vi "Main.vi"(11 "Module Admin":refnum<class "Delacor_lib_QMH_Module Admin.lvclass">) -> ()   [LabVIEW 2021, in "Log.lvlib"]
doc: "This template is based off of the Queued Message Handler design pattern and the Queued Message Handler project template that ships with LabVIEW.\n\nThe main difference is that the queue is private to this module and communication between modules is performed via Broadcast and Request events.\n\nRequest events are wrapped in public API methods and are handled in the Event Handling Loop (EHL) of this VI. Any module can register for Broadcast events sent by this module. The EHL generates messages based on user interface actions.\n\nThe Message Handling Loop (MHL) processes messages generated by the EHL, or by other messages. The messages are string values, so new messages can be added easily to the Message Cases case structure in the MHL. Each message cluster can also provide an optional value for Message Data, which is a variant that can be converted to whatever message-specific data is required.\n_____\nBased on DQMH Project Template 7.0.1.1316."
uses:
  Log.lvlib
  <vilib>/Delacor/Delacor QMH/Libraries/Module Admin_class/Delacor_lib_QMH_Module Admin.lvclass
  Module Data--cluster.ctl
  <vilib>/Delacor/Delacor QMH/Libraries/Message Queue_class/Delacor_lib_QMH_Message Queue.lvclass/Delacor_lib_QMH_Message Queue.ctl
  Stop Argument--cluster.ctl
  <vilib>/Delacor/Delacor QMH/Libraries/Module Admin_class/Delacor_lib_QMH_Module Admin.lvclass/Delacor_lib_QMH_Module Admin.ctl
  Log Start Argument--cluster.ctl
  Log Stop Argument--cluster.ctl
  Log Data Argument--cluster.ctl
  <vilib>/Utility/miscctls.llb/LVPointTypeDef.ctl
  <vilib>/Delacor/Delacor QMH/Libraries/Message Queue_class/Delacor_lib_QMH_Enqueue Message (Single).vi
  <vilib>/Delacor/Delacor QMH/Libraries/Module Admin_class/Delacor_lib_QMH_Get External Launch.vi
  <vilib>/Delacor/Delacor QMH/Libraries/Message Queue_class/Delacor_lib_QMH_Message Queue.lvclass
panel:
  out "error out":errorcluster
  out "Status":string
  in  "Simulate MHL Error":bool
  in  "Simulate EHL Error":bool
  # "Other processes communicate with this Module via its Public API (wrappers for its Request Events).\n\nThis Module communicates with other processes via its Broadcast Events.\nAny process that wants to receive these messages can register for this module's Broadcast events."
  # "This template is for the DQMH framework. See the block diagram for more information on how to use this template."
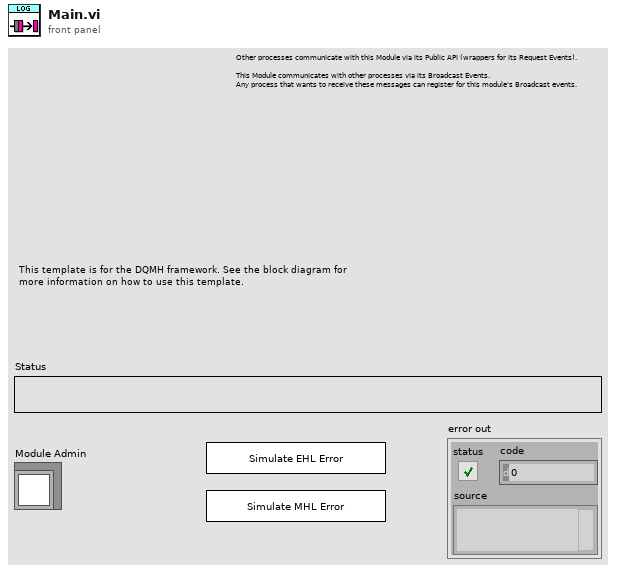
[diagram p1: front panel]
types:
  T1 = typedef "Log.lvlib/Request Events--cluster.ctl" = cluster{"Stop Module":refnum<user-event>, "Show Panel":refnum<user-event>, "Hide Panel":refnum<user-event>, "Get Module Execution Status":refnum<user-event>, "Show Diagram":refnum<user-event>, "Log Start":refnum<user-event>, "Log Stop":refnum<user-event>, "Log Data":refnum<user-event>}
  T2 = typedef "Log.lvlib/Module Data--cluster.ctl" = cluster{"Status":string, "Signal Name":string, "Log Status":bool, "Log Reference":refnum<k34>}
  T3 = enum32{"invalid lock state", "Not Locked", "Locked (No Password)", "Password-protected"}
  T4 = typedef "Log.lvlib/Stop Argument--cluster.ctl" = cluster{"Origin":string, "Exit via Stop Module Req?":bool, "Wait for Module to stop?":bool}
  T5 = typedef "Log.lvlib/Log Start Argument--cluster.ctl" = cluster{"Signal Name":string}
  T6 = typedef "Log.lvlib/Log Stop Argument--cluster.ctl" = cluster{"Boolean":bool}
  T7 = typedef "Log.lvlib/Log Data Argument--cluster.ctl" = cluster{"Signal":waveform(dbl)}
  T8 = typedef "LVPointTypeDef.ctl" = cluster{"Horizontal":i16, "Vertical":i16}
  T9 = enum32{"Invalid", "Standard", "Closed", "Hidden", "Minimized", "Maximized"}
  T10 = enum16{"open", "open or create", "create or replace", "create", "open (read-only)"}
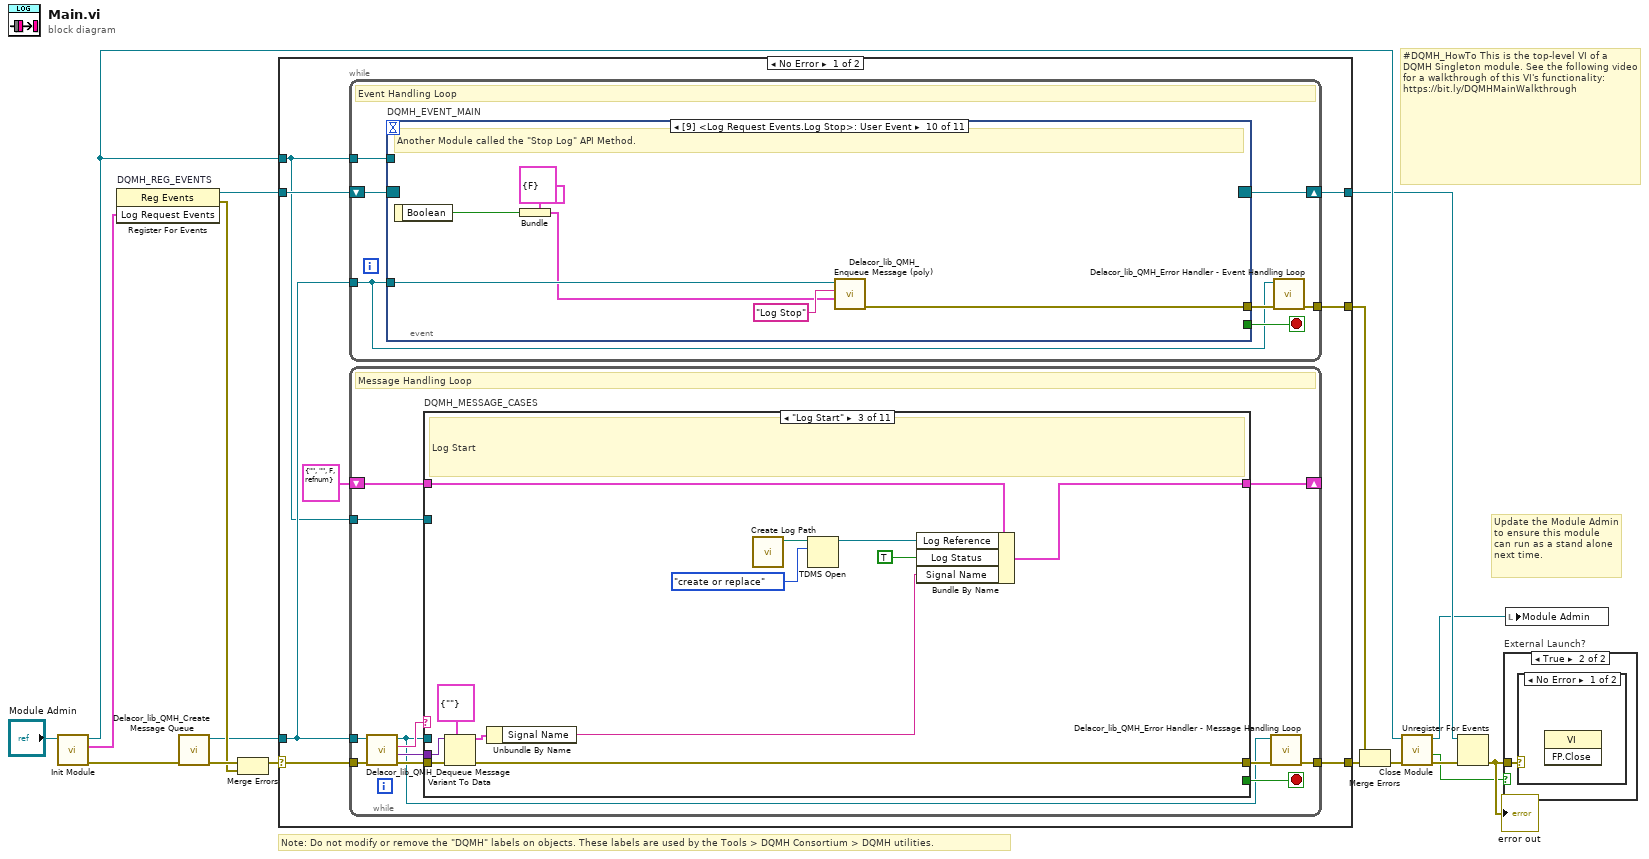
[diagram p0: block diagram]
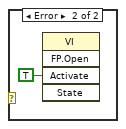
[diagram p3: hidden frame]
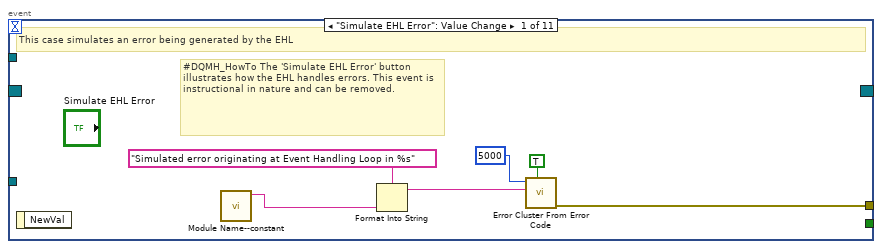
[diagram p4: hidden frame]
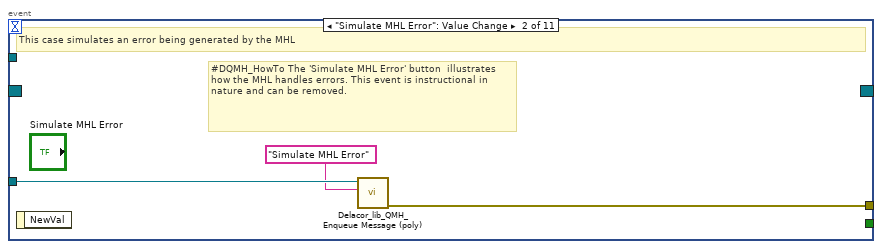
[diagram p5: hidden frame]
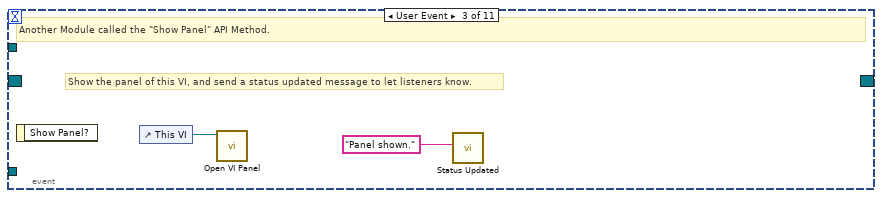
[diagram p6: hidden frame]
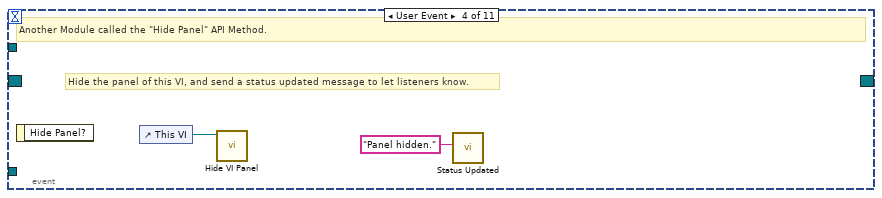
[diagram p7: hidden frame]
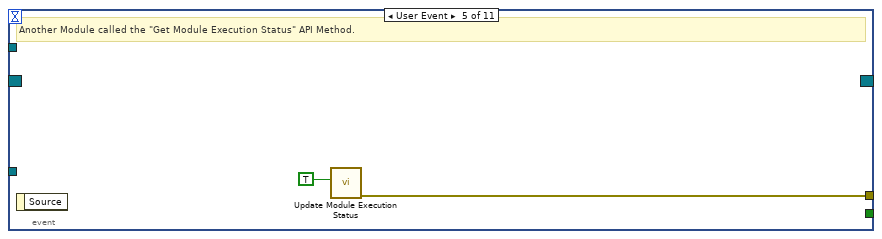
[diagram p8: hidden frame]
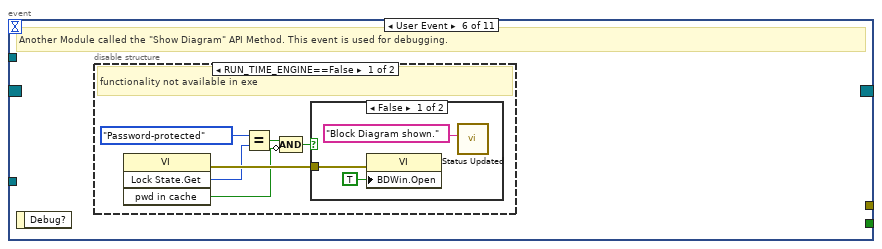
[diagram p9: hidden frame]
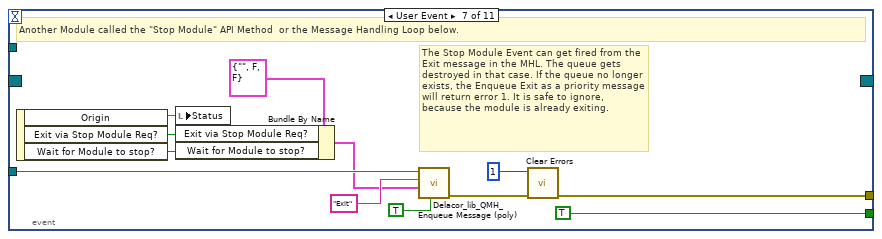
[diagram p12: hidden frame]
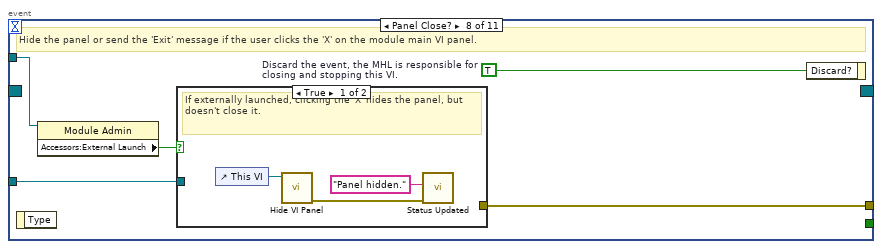
[diagram p13: hidden frame]
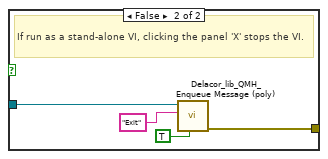
[diagram p14: hidden frame]
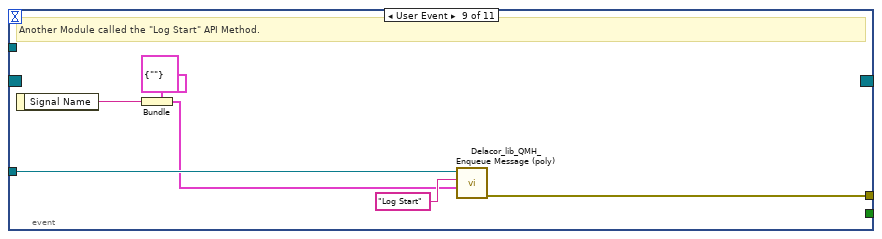
[diagram p15: hidden frame]
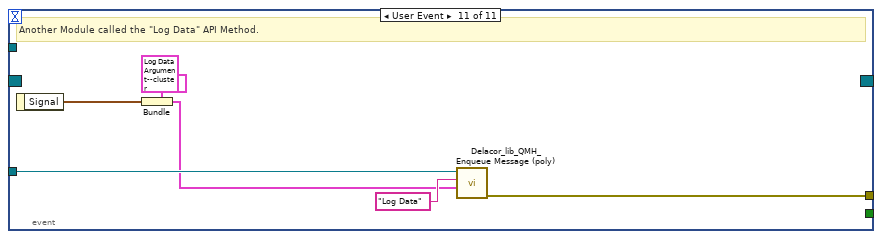
[diagram p16: hidden frame]
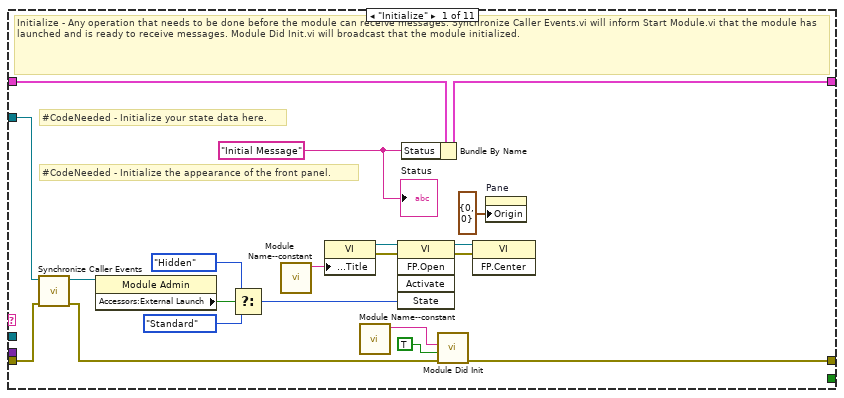
[diagram p17: hidden frame]
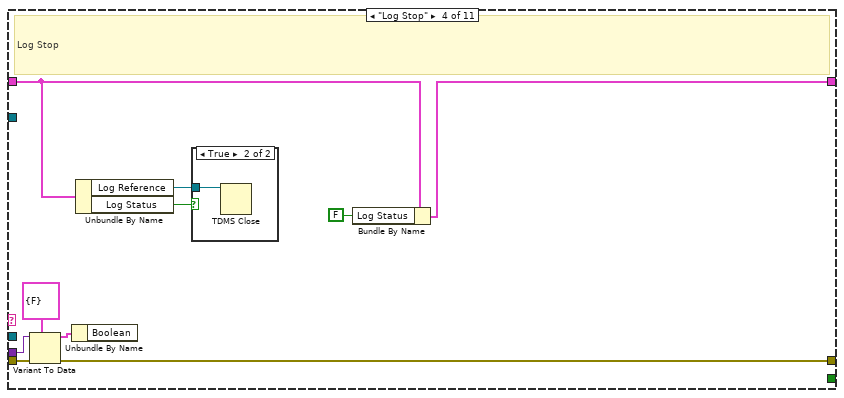
[diagram p19: hidden frame]
diagram:
  # "#DQMH_HowTo This is the top-level VI of a DQMH Singleton module. See the following video for a walkthrough of this VI's functionality: https://bit.ly/DQMHMainWalkthrough"
  # "Note: Do not modify or remove the \"DQMH\" labels on objects. These labels are used by the Tools > DQMH Consortium > DQMH utilities."
  # "Update the Module Admin to ensure this module can run as a stand alone next time."
  n1 = call "Init Module.vi"("Singleton Module Admin in"="Module Admin") -> ("error out"=w16:errorcluster, "Log Request Events"=w5:T1, "Singleton Module Admin out"=w8:refnum<class "Delacor_lib_QMH_Module Admin.lvclass">)  [unwired: 8 in]
  n2 = register-events "DQMH_REG_EVENTS"(w5) -> (reference out=w6:refnum<event-registration>, error out=w9:errorcluster)  [unwired: 2 in]
  n3 = call <vilib>:"Delacor_lib_QMH_Create Message Queue.vi"("error in"=w16) -> ("error out"=w11:errorcluster, "Message Queue"=w4:refnum<class "Delacor_lib_QMH_Message Queue.lvclass">)  [unwired: 9 in]
  n4 = Merge Errors(w11, w9) -> (w10:errorcluster)
  n5 = case shown="No Error" w10 {
    selector: w10 -> [w23 w233]
    tunnel: [w25 w232] -> w17
    tunnel: [w22 w231] -> w7
    tunnel: w6 -> [w20 w231]
    tunnel: w4 -> [w19 w226]
    tunnel: [w24 _] -> w14
    tunnel: w8 -> [w18 w227]
    frame No Error {
      n6 = while {
        tunnel: w19 -> [w26]
        shift-right: [w29] -> w22
        shift-left: w20 -> [w30]
        tunnel: [w31] -> w24
        tunnel: w18 -> [w27]
        stop <- w28 stop-if-true
        # "Event Handling Loop"
        n7 = event "DQMH_EVENT_MAIN" shown="[9] <Log Request Events.Log Stop>: User Event" {
          selector: w30 -> [_ _ _ _ _ _ _ _ _ _ _]
          dyn-events: [_ _ _ _ _ _ _ _ _ _ _] -> w29
          timeout: _ -> [_ _ _ _ _ _ _ _ _ _ _]
          tunnel: [_ _ _ _ _ _ TRUE ("Discard?") _ _ _ _] -> w28
          tunnel: w26 -> [_ w40 _ _ _ _ w64 w71 w86 w92 w98]
          tunnel: [w38 w41 _ _ w47 _ w67 w73 w81 w87 w93] -> w32
          tunnel: w27 -> [_ _ _ _ _ _ _ w70 _ _ _]
          event "Simulate EHL Error": Value Change {
            # "#DQMH_HowTo The 'Simulate EHL Error' button  illustrates how the EHL handles errors. This event is instructional in nature and can be removed."
            # "This case simulates an error being generated by the EHL"
            n8 = event-data() -> ()  [unwired: 1 in, 1 out]
            n9 = call "Module Name--constant.vi"() -> ("Module Name"=w35:string)  [unwired: 11 in]
            n10 = Format Into String(format string="Simulated error originating at Event Handling Loop in %s", w35) -> (resulting string=w36:string)  [unwired: 2 in, 1 out]
            n11 = call <vilib>:"Error Cluster From Error Code.vi"("show call chain? (False)"=TRUE, "error message (\"\")"=w36, "error code (0)"=5000) -> ("error out"=w38:errorcluster)  [unwired: 6 in]
          }
          event "Simulate MHL Error": Value Change {
            # "#DQMH_HowTo The 'Simulate MHL Error' button  illustrates how the MHL handles errors. This event is instructional in nature and can be removed."
            # "This case simulates an error being generated by the MHL"
            n12 = event-data() -> ()  [unwired: 1 in, 1 out]
            n13 = call-poly <vilib>:"Delacor_lib_QMH_Enqueue Message (poly).vi"("Message"="Simulate MHL Error", "Message Queue in"=w40) -> ("error out"=w41:errorcluster)  [unwired: 8 in, 1 out]
          }
          event User Event {
            # "Show the panel of this VI, and send a status updated message to let listeners know."
            # "Another Module called the \"Show Panel\" API Method."
            n14 = event-data() -> ()  [unwired: 1 in, 1 out]
            n15 = control-ref of="This VI"() -> (w43:refnum<vi>)
            n16 = call "Open VI Panel.vi"("VI"=w43) -> ()  [unwired: 10 in, 1 out]
            n17 = call "Status Updated.vi"("Status"="Panel shown." ("format string")) -> ()  [unwired: 10 in, 1 out]
          }
          event User Event {
            # "Hide the panel of this VI, and send a status updated message to let listeners know."
            # "Another Module called the \"Hide Panel\" API Method."
            n18 = event-data() -> ()  [unwired: 1 in, 1 out]
            n19 = control-ref of="This VI"() -> (w45:refnum<vi>)
            n20 = call "Hide VI Panel.vi"("VI"=w45) -> ()  [unwired: 10 in, 1 out]
            n21 = call "Status Updated.vi"("Status"="Panel hidden." ("format string")) -> ()  [unwired: 10 in, 1 out]
          }
          event User Event {
            # "Another Module called the \"Get Module Execution Status\" API Method."
            n22 = event-data() -> ()  [unwired: 1 in, 1 out]
            n23 = call "Update Module Execution Status.vi"("Running?"=TRUE) -> ("error out"=w47:errorcluster)  [unwired: 10 in]
          }
          event User Event {
            # "Another Module called the \"Show Diagram\" API Method. This event is used for debugging."
            n24 = event-data() -> ()  [unwired: 1 in, 1 out]
            n25 = disable-structure shown="RUN_TIME_ENGINE==False" {
              frame condition #0 (active) {
                # "functionality not available in exe"
                n26 = invoke on="Invoke Node" class="VI" method="Lock State.Get"() -> (error out=w53:errorcluster, "Get Lock State"=w52:T3, "pwd in cache"=w49:bool)  [unwired: 4 in, 1 out]
                n27 = Equal?(x=T3."Password-protected", y=w52) -> (x = y?=w50:bool)
                n28 = Compound Arithmetic op=AND(w50, invert w49) -> (w48:bool)
                n29 = case shown="False" w48 {
                  tunnel: w53 -> [w56 _]
                  frame False {
                    n30 = property on="Property Node" class="VI"(error in=w56, "BDWin.Open"=TRUE ("Block Diagram Window:Open")) -> ()  [unwired: 1 in, 2 out]
                    n31 = call "Status Updated.vi"("Status"="Block Diagram shown." ("format string")) -> ()  [unwired: 10 in, 1 out]
                  }
                  frame True {
                    # "Password-protected VI, and the password is not in the cache. Do not show the diagram."
                  }
                }
              }
              frame condition #1 {
              }
            }
          }
          event User Event {
            # "The Stop Module Event can get fired from the Exit message in the MHL. The queue gets destroyed in that case. If the queue no longer exists, the Enqueue Exit as a priority message will return error 1. It is safe to ignore, because the module is already exiting."
            # "Another Module called the \"Stop Module\" API Method  or the Message Handling Loop below."
            n32 = event-data() -> ("Origin"=w63:string, "Exit via Stop Module Req?"=w59:bool, "Wait for Module to stop?"=w58:bool)  [unwired: 1 in]
            n33 = local write "Status"(w63) -> ()
            n34 = Bundle By Name(cluster=T4 {"Origin"="", "Exit via Stop Module Req?"=FALSE, "Wait for Module to stop?"=FALSE} ("Stop Argument"), "Exit via Stop Module Req?"=w59, "Wait for Module to stop?"=w58) -> (w57:T4)
            n35 = call-poly <vilib>:"Delacor_lib_QMH_Enqueue Message (poly).vi"("Priority Message? (F)"=TRUE, "Message Data"=w57, "Message"="Exit", "Message Queue in"=w64) -> ("error out"=w68:errorcluster)  [unwired: 6 in, 1 out]
            n36 = call <vilib>:"Clear Errors.vi"("error in (no error)"=w68, "specific error code to clear (0: all)"=1) -> ("error out"=w67:errorcluster)  [unwired: 4 in, 1 out]
          }
          event Panel Close? {
            w72 = TRUE  # Discard the event, the MHL is responsible for closing and stopping this VI.
            # "Hide the panel or send the 'Exit' message if the user clicks the 'X' on the module main VI panel."
            n37 = event-data() -> ()  [unwired: 1 in, 1 out]
            n38 = property on="Property Node" class="Module Admin"(reference=w70) -> ("Accessors:External Launch"=w69:bool)  [unwired: 1 in, 2 out]
            n39 = case shown="True" w69 {
              tunnel: w71 -> [_ w79]
              tunnel: [_ w80] -> w73
              frame True {
                # "If externally launched, clicking the 'X' hides the panel, but doesn't close it."
                n40 = control-ref of="This VI"() -> (w76:refnum<vi>)
                n41 = call "Hide VI Panel.vi"("VI"=w76) -> ("error out"=w74:errorcluster)  [unwired: 10 in]
                n42 = call "Status Updated.vi"("error in"=w74, "Status"="Panel hidden." ("format string")) -> ()  [unwired: 9 in, 1 out]
              }
              frame False {
                # "If run as a stand-alone VI, clicking the panel 'X' stops the VI."
                n43 = call-poly <vilib>:"Delacor_lib_QMH_Enqueue Message (poly).vi"("Priority Message? (F)"=TRUE, "Message"="Exit", "Message Queue in"=w79) -> ("error out"=w80:errorcluster)  [unwired: 7 in, 1 out]
              }
            }
            n44 = event-data ("Event Filter Node")("Discard?"=w72) -> ()  [unwired: 1 in, 1 out]
          }
          event User Event {
            # "Another Module called the \"Log Start\" API Method."
            n45 = event-data() -> ("Signal Name"=w82:string)  [unwired: 1 in]
            n46 = Bundle(cluster=T5 {"Signal Name"=""} ("Log Start Argument"), "Signal Name"=w82) -> (w83:T5)
            n47 = call-poly <vilib>:"Delacor_lib_QMH_Enqueue Message (poly).vi"("Message Data"=w83, "Message"="Log Start", "Message Queue in"=w86) -> ("error out"=w81:errorcluster)  [unwired: 7 in, 1 out]
          }
          event User Event {
            # "Another Module called the \"Stop Log\" API Method."
            n48 = event-data() -> ("Boolean"=w88:bool)  [unwired: 1 in]
            n49 = Bundle(cluster=T6 {"Boolean"=FALSE} ("Stop Log Argument"), "Boolean"=w88) -> (w89:T6)
            n50 = call-poly <vilib>:"Delacor_lib_QMH_Enqueue Message (poly).vi"("Message Data"=w89, "Message"="Log Stop", "Message Queue in"=w92) -> ("error out"=w87:errorcluster)  [unwired: 7 in, 1 out]
          }
          event User Event {
            # "Another Module called the \"Log Data\" API Method."
            n51 = event-data() -> ("Signal"=w94:waveform(dbl))  [unwired: 1 in]
            n52 = Bundle(cluster=T7 {"Signal"={"t0"=timestamp(0 s since 1904-01-01), "dt"=1.0, "Y"=[]}} ("Log Data Argument"), "Signal"=w94) -> (w95:T7)
            n53 = call-poly <vilib>:"Delacor_lib_QMH_Enqueue Message (poly).vi"("Message Data"=w95, "Message"="Log Data", "Message Queue in"=w98) -> ("error out"=w93:errorcluster)  [unwired: 7 in, 1 out]
          }
        }
        n54 = call-dynamic "Delacor_lib_QMH_Error Handler - Event Handling Loop.vi"("error in"=w32, "Message Queue in"=w26) -> ("dup error in"=w31:errorcluster)  [unwired: 8 in, 1 out]
      }
      n55 = while {
        tunnel: w19 -> [w99]
        shift-right: [w107] -> _
        shift-left: T2 {"Status"="", "Signal Name"="", "Log Status"=FALSE, "Log Reference"=refnum} ("Data Cluster") -> [w108]
        tunnel: w23 -> [w110]
        tunnel: [w102] -> w25
        tunnel: w18 -> [w103]
        stop <- w106 stop-if-true
        # "Message Handling Loop"
        n56 = call-dynamic "Delacor_lib_QMH_Dequeue Message.vi"("error in"=w110, "Message Queue in"=w99) -> ("error out"=w109:errorcluster, "Message Data"=w104:variant, "Message"=w105:string, "Message Queue out"=w100:refnum<class "Delacor_lib_QMH_Message Queue.lvclass">)  [unwired: 6 in]
        n57 = case "DQMH_MESSAGE_CASES" shown="\"Log Start\"" w105 {
          selector: w105 -> [_ _ _ _ _ _ _ _ _ _ w221]
          tunnel: w100 -> [_ _ _ _ _ _ _ _ w187 w209 _]
          tunnel: w109 -> [w128 w132 w144 w154 w165 w172 w174 w183 w194 w215 w224]
          tunnel: [w126 w132 w143 w153 w164 w171 w174 w182 w190 w210 w225] -> w101
          tunnel: w108 -> [w117 w131 w139 w147 w160 w170 w173 w180 w189 w208 w222]
          tunnel: [w116 w131 w136 w148 w160 w170 w173 w180 w189 w208 w222] -> w107
          tunnel: [_ _ _ _ _ _ _ _ _ w207 _] -> w106
          tunnel: w104 -> [_ _ w142 w152 w163 _ _ _ w188 w206 _]
          tunnel: w103 -> [w118 _ _ _ _ _ _ _ w186 w201 _]
          frame "Initialize" {
            w112 = "Initial Message" ("Initial Message")
            # "#CodeNeeded - Initialize the appearance of the front panel."
            # "#CodeNeeded - Initialize your state data here."
            # "Initialize - Any operation that needs to be done before the module can receive messages. Synchronize Caller Events.vi will inform Start Module.vi that the module has launched and is ready to receive messages. Module Did Init.vi will broadcast that the module initialized."
            n58 = call "Synchronize Caller Events.vi"("error in"=w128, "Singleton Module Admin in"=w118) -> ("error out"=w127:errorcluster, "Singleton Module Admin out"=w113:refnum<class "Delacor_lib_QMH_Module Admin.lvclass">)  [unwired: 8 in]
            n59 = property on="Property Node" class="Module Admin"(reference=w113) -> ("Accessors:External Launch"=w122:bool)  [unwired: 1 in, 2 out]
            n60 = Select(t=T9."Hidden" ("State"), s=w122, f=T9."Standard" ("State")) -> (s? t:f=w119:T9)
            n61 = call "Module Name--constant.vi"() -> ("Module Name"=w125:string)  [unwired: 11 in]
            n62 = property on="Property Node" class="VI"("Front Panel.Title"=w125) -> (reference out=w124:refnum<vi>, error out=w130:errorcluster)  [unwired: 2 in]
            n63 = call "Module Name--constant.vi"() -> ("Module Name"=w114:string)  [unwired: 11 in]
            n64 = invoke on="Invoke Node" class="VI" method="FP.Open"(reference=w124, error in=w130, "State"=w119) -> (reference out=w123:refnum<vi>, error out=w129:errorcluster)  [unwired: 2 in, 3 out]
            n65 = Bundle By Name(cluster=w117, "Status"=w112) -> (w116:T2)
            n66 = call "Module Did Init.vi"("error in"=w127, "Initialized?"=TRUE, "Origin"=w114) -> ("error out"=w126:errorcluster)  [unwired: 8 in]
            n67 = invoke on="Invoke Node" class="VI" method="FP.Center"(reference=w123, error in=w129) -> ()  [unwired: 1 in, 3 out]
            n68 = property on="Pane" class="Pane"("Origin"=T8 {"Horizontal"=0, "Vertical"=0}) -> ()  [unwired: 2 in, 2 out]
            "Status" <- w112
          }
          frame "---Module Specific---" {
            # "Separator -- The following cases handle messages specific to this Module."
          }
          frame "Log Start" {
            # "Log Start"
            n69 = Variant To Data(error in=w144, type=T5 {"Signal Name"=""} ("Log Start Argument"), Variant=w142) -> (data=w140:T5, error out=w143:errorcluster)
            n70 = Unbundle By Name(w140) -> ("Signal Name"=w137:string)
            n71 = call "Create Log Path.vi"() -> ("log path"=w135:path)  [unwired: 11 in]
            n72 = TDMS Open(10:T10."create or replace" ("operation (0:open)"), 11:w135) -> (3:w133:refnum<k34>)  [unwired: 5 in, 1 out]
            n73 = Bundle By Name(cluster=w139, "Log Reference"=w133, "Log Status"=TRUE, "Signal Name"=w137) -> (w136:T2)
          }
          frame "Log Stop" {
            # "Log Stop"
            n74 = Variant To Data(error in=w154, type=T6 {"Boolean"=FALSE} ("Stop Log Argument"), Variant=w152) -> (data=w150:T6, error out=w153:errorcluster)
            n75 = Unbundle By Name(w150) -> ()  [unwired: 1 out]
            n76 = Unbundle By Name(w147) -> ("Log Reference"=w146:refnum<k34>, "Log Status"=w145:bool)
            n77 = case shown="True" w145 {
              tunnel: w146 -> [_ w155]
              frame False {
              }
              frame True {
                n78 = TDMS Close(11:w155) -> ()  [unwired: 1 in, 2 out]
              }
            }
            n79 = Bundle By Name(cluster=w147, "Log Status"=FALSE) -> (w148:T2)
          }
          frame "Log Data" {
            # "Log Data"
            n80 = Variant To Data(error in=w165, type=T7 {"Signal"={"t0"=timestamp(0 s since 1904-01-01), "dt"=1.0, "Y"=[]}} ("Log Data Argument"), Variant=w163) -> (data=w161:T7, error out=w164:errorcluster)
            n81 = Unbundle By Name(w161) -> ("Signal"=w158:waveform(dbl))
            n82 = Unbundle By Name(w160) -> ("Log Reference"=w159:refnum<k34>, "Signal Name"=w157:string, "Log Status"=w156:bool)
            n83 = case shown="True" w156 {
              tunnel: w159 -> [_ w169]
              tunnel: w158 -> [_ w167]
              tunnel: w157 -> [_ w166]
              frame False {
              }
              frame True {
                n84 = TDMS Write(0:w169, 5:"signal" ("group name in (Untitled)"), 7:w166, 9:w167) -> ()  [unwired: 2 in, 4 out]
              }
            }
          }
          frame "---Copy This Frame---" {
            # "Duplicate this frame when creating new messages.  Change this comment in the duplicated frame to describe this message."
            n85 = Merge Errors(w172) -> (w171:errorcluster)
          }
          frame "---Exit and Error Handling---" {
            # "Separator - The following cases handle errors and exit messages."
          }
          frame "Simulate MHL Error" {
            # "#DQMH_HowTo The 'Simulate MHL Error' button  illustrates how the MHL handles errors. This event is instructional in nature and can be removed."
            # "Simulate an error occurring at the MHL"
            n86 = call "Module Name--constant.vi"() -> ("Module Name"=w176:string)  [unwired: 11 in]
            n87 = Format Into String(format string="Simulated error originating at Message Handling Loop in %s", w176) -> (resulting string=w177:string)  [unwired: 2 in, 1 out]
            n88 = call <vilib>:"Error Cluster From Error Code.vi"("show call chain? (False)"=TRUE, "error message (\"\")"=w177, "error code (0)"=5001) -> ("error out"=w181:errorcluster)  [unwired: 6 in]
            n89 = Merge Errors(w183, w181) -> (w182:errorcluster)
          }
          frame "Error" {
            # "#CodeRecommended - If the module is running in standalone mode (External Launch = FALSE), this code will pop up an error dialog and call the 'Exit' message if an error occurs. Add more fine-grained error management here."
            # "Error - Check the error message data and respond accordingly. This message is sent by the \"Error Handler\" VIs at the end of each loop in this application."
            n90 = property on="Property Node" class="Module Admin"(reference=w186) -> ("Accessors:External Launch"=w185:bool)  [unwired: 1 in, 2 out]
            n91 = Variant To Data(error in=w194, type=errorcluster {"status"=FALSE, "code"=0, "source"=""} ("error constant"), Variant=w188) -> (data=w184:errorcluster, error out=w192:errorcluster)
            n92 = local write "error out"(w184) -> ()
            n93 = call "Error Reported.vi"("Error"=w184) -> ()  [unwired: 10 in, 1 out]
            n94 = case shown="False" w185 {
              tunnel: [w199 _] -> w191
              tunnel: w187 -> [w197 _]
              tunnel: w184 -> [w198 _]
              frame False {
                n95 = disable-structure shown="Default" {
                  disable-tunnel: w198 -> [w200 _]
                  frame condition #0 (active) {
                    # "If the module is running standalone, then pop up an error dialog and call the \"Exit\" message."
                    n96 = call <vilib>:"Simple Error Handler.vi"("error in (no error)"=w200) -> ()  [unwired: 4 in, 5 out]
                  }
                  frame condition #1 {
                    # "To prevent the Simple Error Handler VI from being loaded (e.g. when deploying to a Real-Time target), add the Conditional Disable Symbol \"DQMH_Disable_SEH\" to your project and set it to TRUE."
                  }
                }
                n97 = call-poly <vilib>:"Delacor_lib_QMH_Enqueue Message (poly).vi"("Priority Message? (F)"=TRUE, "Message"="Exit", "Message Queue in"=w197) -> ("error out"=w199:errorcluster)  [unwired: 7 in, 1 out]
              }
              frame True {
                # "If the module was launched externally, calling the Error Reported broadcast VI is the only action performed by the \"Error\" message. The module's caller can then process the error appropriately."
              }
            }
            n98 = Merge Errors(w192, w191) -> (w190:errorcluster)
          }
          frame "Exit" {
            w205 = 91  # 91: not all Exit messages will have an argument
            w207 = TRUE  # Stop the VI
            # "Release the message queue reference"
            # "#CodeNeeded - Add any required cleanup code here."
            # "Exit - Exit the application."
            n99 = Variant To Data(error in=w215, type=T4 {"Origin"="", "Exit via Stop Module Req?"=FALSE, "Wait for Module to stop?"=FALSE} ("Stop Argument"), Variant=w206) -> (data=w203:T4, error out=w212:errorcluster)
            n100 = call <vilib>:"Clear Errors.vi"("error in (no error)"=w212, "specific error code to clear (0: all)"=w205) -> ("error out"=w214:errorcluster)  [unwired: 4 in, 1 out]
            n101 = control-ref of="This VI"() -> (w202:refnum<vi>)
            n102 = call-dynamic "Delacor_lib_QMH_Release Message Queue.vi"("error in"=w214, "Message Queue"=w209) -> ("error out"=w213:errorcluster)  [unwired: 9 in]
            n103 = call "Handle Exit.vi"("Stop Argument"=w203, "Admin in"=w201, "VI reference"=w202) -> ("error out"=w211:errorcluster)  [unwired: 7 in, 1 out]
            n104 = Merge Errors(w213, w211) -> (w210:errorcluster)
            n105 = call "Error Reported.vi"("Error"=w210) -> ()  [unwired: 10 in, 1 out]
          }
          frame Default {
            # "'Default' case only runs if there is a message that isn't defined in any of the other cases.  Output a programming error."
            n106 = call "Module Name--constant.vi"() -> ("Module Name"=w220:string)  [unwired: 11 in]
            n107 = Format Into String(format string="The invalid message string \"%s\" was received in the Message Handling Loop for module \"%s\".", w221, w220) -> (resulting string=w216:string)  [unwired: 2 in, 1 out]
            n108 = call <vilib>:"Error Cluster From Error Code.vi"("show call chain? (False)"=TRUE, "error message (\"\")"=w216, "error code (0)"=1) -> ("error out"=w223:errorcluster)  [unwired: 6 in]
            n109 = Merge Errors(w224, w223) -> (w225:errorcluster)
          }
        }
        n110 = call-dynamic "Delacor_lib_QMH_Error Handler - Message Handling Loop.vi"("error in"=w101, "Message Queue in"=w100) -> ("dup error in"=w102:errorcluster)  [unwired: 8 in, 1 out]
      }
    }
    frame Error {
      # "Synchronize Caller Events.vi will inform Start Module.vi that the module has launched and will let the code calling Start Module.vi register for broadcasts and would permit the caller receive the broadcast that an error occurred at launch time."
      n111 = call-dynamic "Delacor_lib_QMH_Release Message Queue.vi"("error in"=w233, "Message Queue"=w226) -> ("error out"=w232:errorcluster)  [unwired: 9 in]
      n112 = call "Synchronize Caller Events.vi"("Singleton Module Admin in"=w227) -> ("error out"=w234:errorcluster)  [unwired: 9 in, 1 out]
      n113 = call "Module Name--constant.vi"() -> ("Module Name"=w230:string)  [unwired: 11 in]
      n114 = Format Into String(format string="An error occurred during initialization. %s is no longer running.", w230) -> (resulting string=w228:string)  [unwired: 2 in, 1 out]
      n115 = Merge Errors(w232, w234) -> (w235:errorcluster)
      n116 = call "Error Reported.vi"("Additional Information"=w228, "Error"=w235) -> ()  [unwired: 9 in, 1 out]
    }
  }
  n117 = Merge Errors(w14, w17) -> (w13:errorcluster)
  n118 = call "Close Module.vi"("error in"=w13, "Module Admin in"=w8) -> ("error out"=w15:errorcluster, "External Launch"=w1:bool, "Module Admin out"=w2:refnum<class "Delacor_lib_QMH_Module Admin.lvclass">)  [unwired: 7 in]
  n119 = Unregister For Events(event registration refnum=w7, error in=w15) -> (error out=w12:errorcluster)
  "error out" <- w12
  n120 = case "External Launch?" shown="True" w1 {
    tunnel: w12 -> [_ w236]
    frame False {
    }
    frame True {
      n121 = case shown="No Error" w236 {
        frame No Error {
          n122 = invoke on="Invoke Node" class="VI" method="FP.Close"() -> ()  [unwired: 3 in, 3 out]
        }
        frame Error {
          n123 = invoke on="Invoke Node" class="VI" method="FP.Open"("Activate"=TRUE ("Activate?")) -> ()  [unwired: 4 in, 5 out]
        }
      }
    }
  }
  n124 = local write "Module Admin"(w2) -> ()
